vi "DWDT Empty Digital.vi"() -> (1 "digital waveform out":digitalwaveform(waveform)={"t0"=timestamp(0 s since 1904-01-01), "dt"=0.0, "Y"={"transitions"=[], "data"=[]}, "error"={"status"=FALSE, "code"=37421928, "source"=""}})   [LabVIEW 2018]
doc: "Returns an empty digital waveform. Use this constant to initialize shift registers or build digital waveforms."
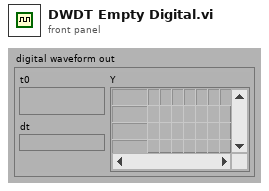
[diagram p1: front panel]
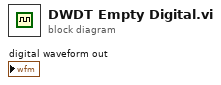
[diagram p0: block diagram]
diagram:
